vi "Constructor.vi"(10 "Capacity":u32) -> (3 "TypedCircularBuffer out":refnum<class "TypedCircularBuffer.lvclass">)   [LabVIEW 2024, in "TypedCircularBuffer.lvclass"]
uses:
  TypedCircularBuffer.lvclass
  TypedCircularBuffer.lvclass/TypedCircularBuffer.ctl
  ReadCount.vi
  Sort.vi
  IsFull.vi
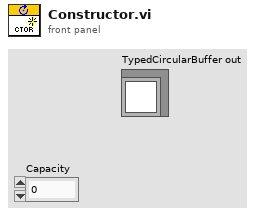
[diagram p1: front panel]
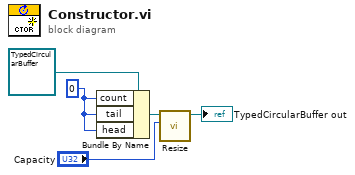
[diagram p0: block diagram]
diagram:
  w3 = u32 0 ("size")
  n1 = Bundle By Name(cluster=refnum<class "TypedCircularBuffer.lvclass"> refnum ("TypedCircularBuffer.lvclass"), "count"=w3, "tail"=w3, "head"=w3) -> (w4:refnum<class "TypedCircularBuffer.lvclass">)
  n2 = call "Resize.vi"("Capacity"="Capacity", "TypedCircularBuffer in"=w4) -> ("TypedCircularBuffer out"=→"TypedCircularBuffer out":refnum<class "TypedCircularBuffer.lvclass">)  [unwired: 9 in]
